vi "toStringArray.vi"(8 "error in (no error)":errorcluster, 11 "RampEvent in":refnum<class "RampEvent.lvclass">) -> (0 "error out":errorcluster, 2 "eventStringArray":string[](array[string]), 3 "RampEvent out":refnum<class "RampEvent.lvclass">)   [LabVIEW 2009, in "Tools.lvlib" / "Scripting.lvlib" / "RampEvent.lvclass"]
uses:
  RampEvent.lvclass
  ScriptEvent.lvclass
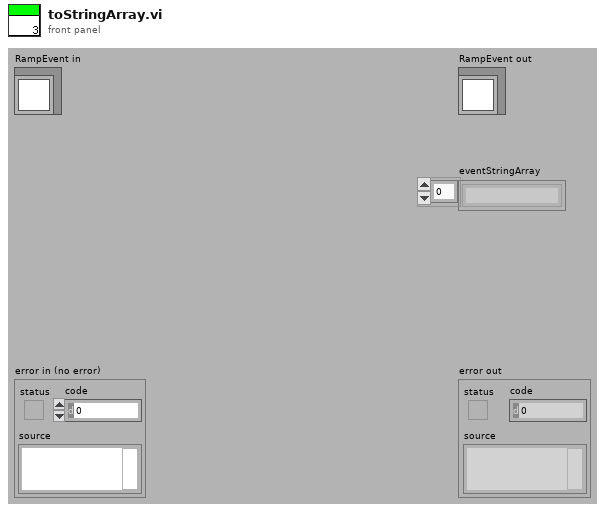
[diagram p1: front panel]
types:
  T1 = cluster{"rampTime":dbl, "timeStep":dbl, "dataValueStep":dbl}
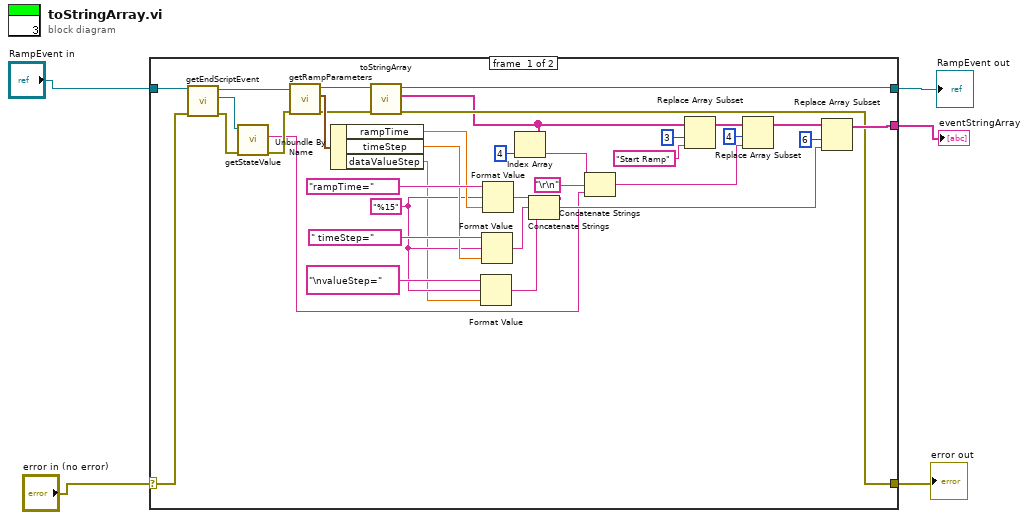
[diagram p0: block diagram]
diagram:
  n1 = case shown="No Error" "error in (no error)" {
    selector: "error in (no error)" -> [w18 w41]
    tunnel: "RampEvent in" -> [w20 w42]
    tunnel: [w40 w42] -> w3
    tunnel: [w24 w41] -> w1
    tunnel: [w25 _] -> w2
    frame #0 {
      w34 = "%15"
      n2 = call "getEndScriptEvent.vi"("error in (no error)"=w18, "RampEvent.lvclass in"=w20) -> ("error out"=w16:errorcluster, "ScriptEvent.lvclass"=w17:refnum<class "ScriptEvent.lvclass">, "RampEvent.lvclass out"=w19:refnum<class "RampEvent.lvclass">)  [unwired: 7 in]
      n3 = call-dynamic "getStateValue.vi"("error in (no error)"=w16, "ScriptEvent in"=w17) -> ("error out"=w15:errorcluster, "stateValue"=w7:string)  [unwired: 7 in, 1 out]
      n4 = call "getRampParameters.vi"("error in (no error)"=w15, "RampEvent in"=w19) -> ("error out"=w21:errorcluster, "RampParameters"=w22:T1, "RampEvent out"=w23:refnum<class "RampEvent.lvclass">)  [unwired: 7 in]
      n5 = Unbundle By Name(w22) -> ("rampTime"=w38:dbl, "timeStep"=w36:dbl, "dataValueStep"=w33:dbl)
      n6 = call-parent "toStringArray.vi"("error in (no error)"=w21, "ScriptEvent in"=w23) -> ("error out"=w24:errorcluster, "eventStringArray"=w11:string[], "ScriptEvent out"=w40:refnum<class "RampEvent.lvclass">)  [unwired: 7 in]
      n7 = Format Value(string ("")="\nvalueStep=", format string=w34, value (0)=w33) -> (output string=w27:string)
      n8 = Format Value(string ("")=" timeStep=", format string=w34, value (0)=w36) -> (output string=w28:string)
      n9 = Format Value(string ("")="rampTime=", format string=w34, value (0)=w38) -> (output string=w29:string)
      n10 = Index Array(array=w11, index=4) -> (element=w9:string)
      n11 = Concatenate Strings(w29, w28, w27) -> (w26:string)
      n12 = Concatenate Strings(w9, "\r\n", w7) -> (w6:string)
      n13 = Replace Array Subset(array=w11, new element="Start Ramp", index=3) -> (w14:string[])
      n14 = Replace Array Subset(array=w14, new element=w6, index=4) -> (w13:string[])
      n15 = Replace Array Subset(array=w13, new element=w26, index=6) -> (w25:string[])
    }
    frame #1 {
    }
  }
  "error out" <- w1
  "RampEvent out" <- w3
  "eventStringArray" <- w2
